vi "Configure Voltage.vi"(8 "error in (no error)":errorcluster, 10 "Voltage":dbl=3.3, 11 "E3631A in":refnum<class "E3631A.lvclass">) -> (0 "error out":errorcluster, 3 "E3631A out":refnum<class "E3631A.lvclass">)   [LabVIEW 2020, in "E3631A.lvclass"]
uses:
  E3631A.lvclass
  C:/Sandbox/RF Bench/Source Code/WiSpry Test Framework/Instruments/Power Supply/Power Supply.lvclass
  C:/Sandbox/RF Bench/Source Code/WiSpry Test Framework/Instruments/Instrument.lvclass
  Instrument.lvclass/Instrument.ctl
  Power Supply.lvclass/Power Supply.ctl
  Instrument.lvclass
  Power Supply.lvclass
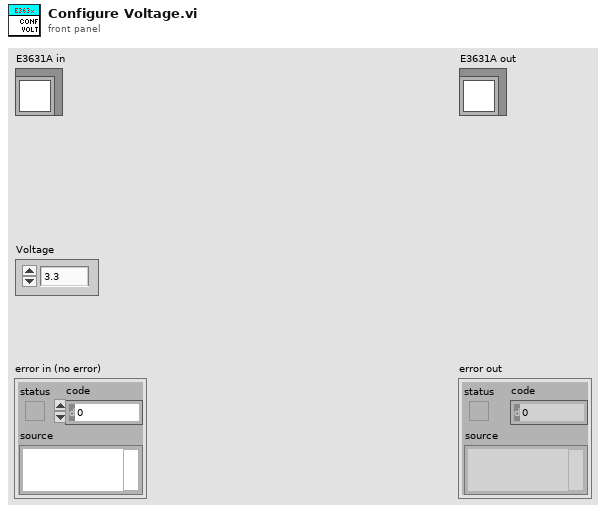
[diagram p1: front panel]
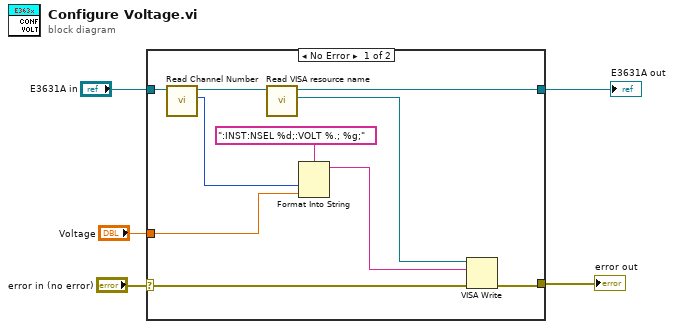
[diagram p0: block diagram]
diagram:
  n1 = case shown="No Error" "error in (no error)" {
    selector: "error in (no error)" -> [w9 w17]
    tunnel: [w15 w17] -> w4
    tunnel: "E3631A in" -> [w8 w16]
    tunnel: [w13 w16] -> w2
    tunnel: "Voltage" -> [w11 _]
    frame No Error {
      n2 = call "Read Channel Number.vi"("Power Supply in"=w8) -> ("Channel Number"=w6:u8, "Power Supply out"=w7:refnum<class "E3631A.lvclass">)  [unwired: 9 in]
      n3 = call "Read VISA resource name.vi"("Instrument in"=w7) -> ("VISA resource name"=w14:refnum<visa-resource-name>, "Instrument out"=w13:refnum<class "E3631A.lvclass">)  [unwired: 9 in]
      n4 = Format Into String(format string=":INST:NSEL %d;:VOLT %.; %g;", w6, w11) -> (resulting string=w10:string)  [unwired: 2 in, 1 out]
      n5 = VISA Write(VISA resource name=w14, write buffer=w10, error in (no error)=w9) -> (error out=w15:errorcluster)  [unwired: 2 out]
    }
    frame Error {
    }
  }
  "error out" <- w4
  "E3631A out" <- w2
